vi "LVClass_ModalCoef ctor Legendre From Slopes.vi"(0 "ModalCoef in":refnum<class "ModalCoef.lvclass">, 5 "HasoSlopes":refnum<class "HasoSlopes.lvclass">, 7 "nb_coefs":u32, 11 "error in (no error)":errorcluster) -> (4 "ModalCoef out":refnum<class "ModalCoef.lvclass">, 15 "error out":errorcluster)   [LabVIEW 2020, in "ModalCoef.lvclass"]
doc: "ModalCoef constructor.\n\n--------------------------------------------------------------------------------\n\n<B>ModalCoefIn </B> : Constant Pointer to ModalCoef object.\n<B>ModalCoefOut </B> : Constant Pointer to ModalCoef object.\n<B>TypePhase </B> : TypePhase Phase mode reconstruction.\n<B>ErrorIn </B> : Error\n<B>ErrorOut </B> : Error\n\n--------------------------------------------------------------------------------"
uses:
  ModalCoef.lvclass
  HasoSlopes.lvclass
  Handle creation.ctl
  ModalCoef.lvclass/ModalCoef.ctl
  LVClass_HasoSlopes Read HasoSlopes _ property.vi
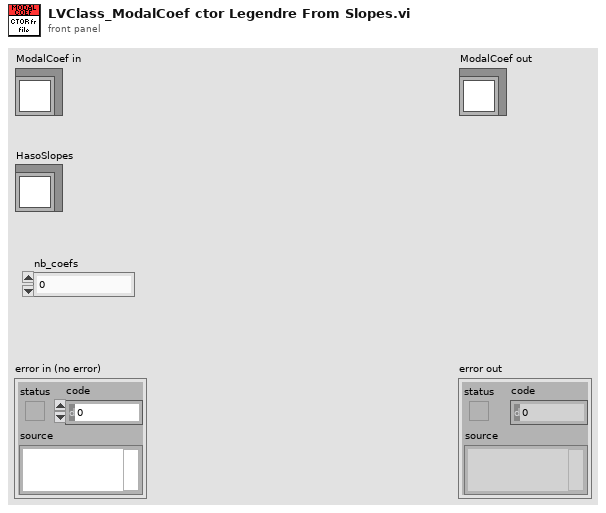
[diagram p1: front panel]
types:
  T1 = typedef "Handle creation.ctl" = enum16{"By ctor", "By write function"}
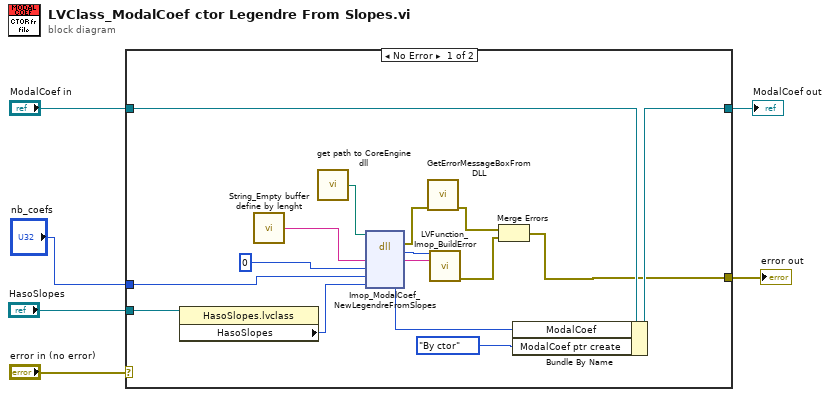
[diagram p0: block diagram]
diagram:
  n1 = case shown="No Error" "error in (no error)" {
    selector: "error in (no error)" -> [_ w24]
    tunnel: [w10 w24] -> w5
    tunnel: [w13 w23] -> w3
    tunnel: "ModalCoef in" -> [w14 w23]
    tunnel: "HasoSlopes" -> [w8 _]
    tunnel: "nb_coefs" -> [w7 _]
    frame No Error {
      n2 = property class="HasoSlopes.lvclass"(reference=w8) -> ("HasoSlopes"=w9:i32)  [unwired: 1 in, 2 out]
      n3 = call "String_Empty buffer define by lenght.vi"() -> ("Empty buffer"=w22:string)  [unwired: 1 in]
      n4 = call "get path to CoreEngine dll.vi"() -> ("path to c_interface_vc100.dll"=w19:path)  [unwired: 12 in, 3 out]
      n5 = dll-call lib="D:/soft/HASO_v3/SVN_trunk/ImOpCoreEngine4_LV2011/DLLs/c_interface_vc100.dll" fn="Imop_ModalCoef_NewLegendreFromSlopes"(path in=w19, "message"=w22, "ModalCoef"=0 ("Pupil"), "nb_coefs"=w7, "Slopes"=w9) -> (error out=w18:errorcluster, "return type"=w20:i32, "message"=w21:string, "ModalCoef"=w16:i32)  [unwired: 4 in, 1 out]
      n6 = call "GetErrorMessageBoxFromDLL.vi"("error IN"=w18) -> ("error OUT"=w12:errorcluster)  [unwired: 10 in]
      n7 = call "LVFunction_Imop_BuildError.vi"("code"=w20, "String to Prepend to source (\"\")"=w21) -> ("error out"=w11:errorcluster)  [unwired: 13 in]
      n8 = Merge Errors(w12, w11) -> (w10:errorcluster)
      n9 = Bundle By Name(cluster=w14, "ModalCoef"=w16, "ModalCoef ptr create"=Handle_creation."By ctor" ("Pupil ptr create")) -> (w13:refnum<class "ModalCoef.lvclass">)
    }
    frame Error {
    }
  }
  "error out" <- w5
  "ModalCoef out" <- w3
